vi "Measure.vi"(8 "error in (no error)":errorcluster, 9 "measurement configuration":variant, 10 "measure call context in":refnum<class "Measure Call Context.lvclass">, 11 "Continuous Counting Mesurement2 in":refnum<class "Continuous Counting Measurement2.lvclass">) -> (0 "error out":errorcluster, 1 "measurement results":variant, 2 "measure call context out":refnum<class "Measure Call Context.lvclass">, 3 "Continuous Counting Mesurement2 out":refnum<class "Continuous Counting Measurement2.lvclass">)   [LabVIEW 2021, in "MeasurementServerTests.lvlib" / "Measurement Service Tests.lvlib" / "Continuous Counting Measurement2.lvclass"]
doc: "Executes the measurement."
uses:
  Continuous Counting Measurement2.lvclass
  Continuous Counting Measurement2.lvclass/Continuous Counting Measurement2.ctl
  Measurement Configuration.ctl
  Runtime/Measurements/Measure Call Context/Measure Call Context.lvclass
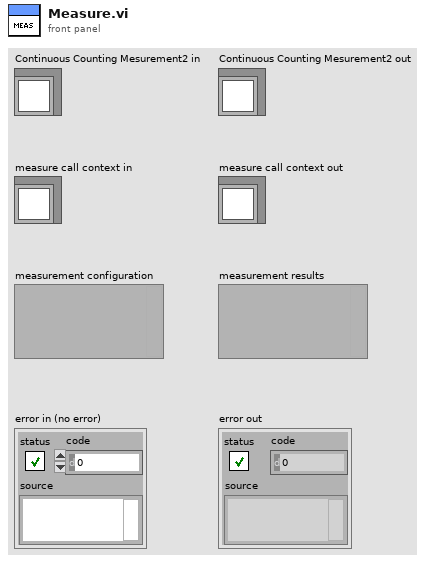
[diagram p1: front panel]
types:
  T1 = typedef "MeasurementServerTests.lvlib/Measurement Service Tests.lvlib/Continuous Counting Measurement2.lvclass/Measurement Configuration.ctl" = cluster{"ms update interval":u32}
  T2 = typedef "MeasurementServerTests.lvlib/Measurement Service Tests.lvlib/Continuous Counting Measurement2.lvclass/Measurement Results.ctl" = cluster{"current count":i64}
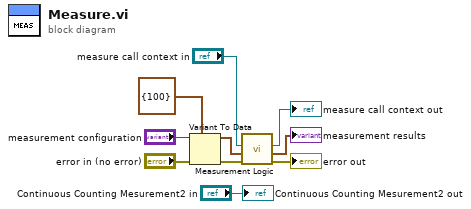
[diagram p0: block diagram]
diagram:
  n1 = Variant To Data(error in="error in (no error)", type=T1 {"ms update interval"=100} ("measurement configuration"), Variant="measurement configuration") -> (data=w2:T1, error out=w6:errorcluster)
  n2 = call "Measurement Logic.vi"("error in"=w6, "measurement configuration"=w2, "measure call context in"="measure call context in") -> ("error out"=→"error out":errorcluster, "measurement results"=→"measurement results":T2, "measure call context out"=→"measure call context out":refnum<class "Measure Call Context.lvclass">)  [unwired: 6 in]
  "Continuous Counting Mesurement2 out" <- "Continuous Counting Mesurement2 in"
